vi "GUIToFMInfo.vi"(0 "carrier frequency":dbl(knob)=10.0 scale=0.0..5000.0, 1 "amplitude":dbl(slide)=1.0 scale=0.0..1.0, 2 "carrier waveform":T2, 3 "modulation frequency":dbl(knob)=10.0 scale=0.0..1000.0, 4 "modulation index":dbl(knob)=1.0 scale=0.0..1.0, 5 "modulator waveform":T2, 6 "sample rate":i32, 7 "buffer size":i32, 8 "bits":i32, 9 "Feedback":bool) -> (16 "FMInfo":T1={"buffer size"=0, "bits"=0, "CarrierInfo"={"frequency"=10.0, "amplitude"=1.0, "sample rate"=0, "waveform type"=enum."Sine"}, "ModulatorInfo"={"frequency"=10.0, "amplitude"=1.0, "sample rate"=0, "waveform type"=enum."Sine"}, "Feedback"=FALSE} {"ModulatorInfo"."amplitude" format="%0.2p"; "ModulatorInfo"."frequency" format="%0.2p"; "CarrierInfo"."amplitude" format="%0.2p"; "CarrierInfo"."frequency" format="%0.2p"})   [LabVIEW 2016]
uses:
  Generation/Oscillator/WaveformType.ctl
  Generation/GenerateWaveform/FMInfo.ctl
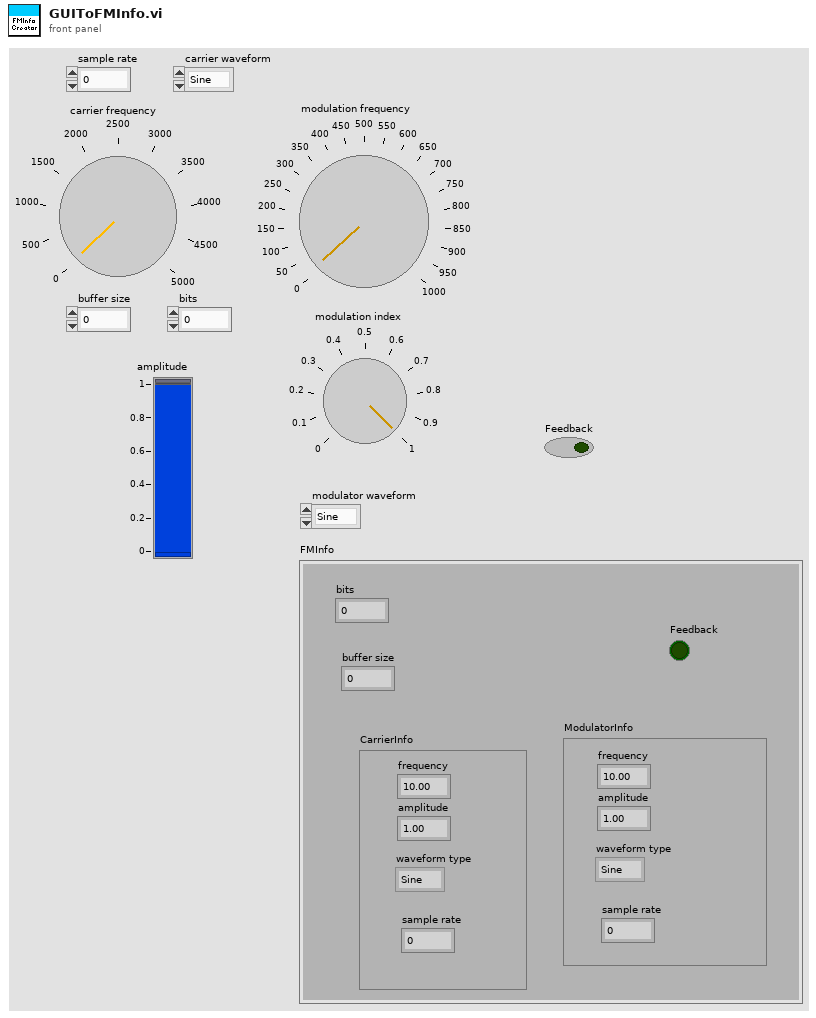
[diagram p1: front panel]
types:
  T1 = typedef "FMInfo.ctl" = cluster{"buffer size":i32, "bits":i32, "CarrierInfo":cluster{"frequency":dbl, "amplitude":dbl, "sample rate":i32, "waveform type":T2}, "ModulatorInfo":cluster{"frequency":dbl, "amplitude":dbl, "sample rate":i32, "waveform type":T2}, "Feedback":bool}
  T2 = typedef "WaveformType.ctl" = enum16{"Sine", "Triangle", "Square", "Sawtooth"}
  T3 = cluster{"frequency":dbl, "amplitude":dbl, "sample rate":i32, "waveform type":T2}
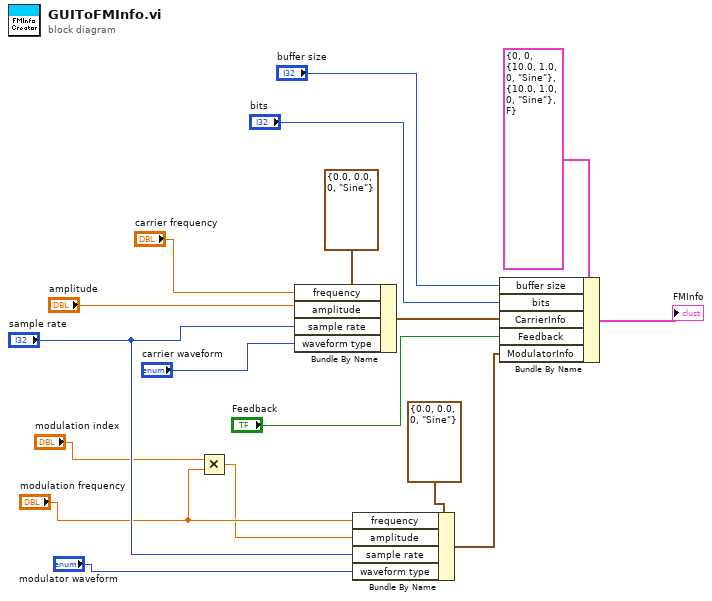
[diagram p0: block diagram]
diagram:
  n1 = Multiply(x="modulation index", y="modulation frequency") -> (x*y=w5:dbl)
  n2 = Bundle By Name(cluster=T3 {"frequency"=0.0, "amplitude"=0.0, "sample rate"=0, "waveform type"=enum."Sine"} ("CarrierInfo"), "frequency"="carrier frequency", "amplitude"="amplitude", "sample rate"="sample rate", "waveform type"="carrier waveform") -> (w16:T3)
  n3 = Bundle By Name(cluster=T3 {"frequency"=0.0, "amplitude"=0.0, "sample rate"=0, "waveform type"=enum."Sine"} ("CarrierInfo"), "frequency"="modulation frequency", "amplitude"=w5, "sample rate"="sample rate", "waveform type"="modulator waveform") -> (w2:T3)
  n4 = Bundle By Name(cluster=T1 {"buffer size"=0, "bits"=0, "CarrierInfo"={"frequency"=10.0, "amplitude"=1.0, "sample rate"=0, "waveform type"=enum."Sine"}, "ModulatorInfo"={"frequency"=10.0, "amplitude"=1.0, "sample rate"=0, "waveform type"=enum."Sine"}, "Feedback"=FALSE} ("FMInfo"), "buffer size"="buffer size", "bits"="bits", "CarrierInfo"=w16, "Feedback"="Feedback", "ModulatorInfo"=w2) -> (→"FMInfo":T1)
